vi "Slider (Main).vi"(6 "Playback":bool, 8 "Slider":i16(slide) scale=0.0..10.0, 10 "Stop":bool, 11 "Error in":errorcluster) -> (15 "Error out":errorcluster)   [LabVIEW 2020]
doc: "This system is used to playback the previous data which is needed to be plotted in the chart and the current value will also be plotted"
uses:
  Typedefs/Cluster data.ctl
panel:
  # "Dynamic and User Events"
  # "Click this button to play the previous value \nrecorded"
  # "Click this button to stop the execution of the VI"
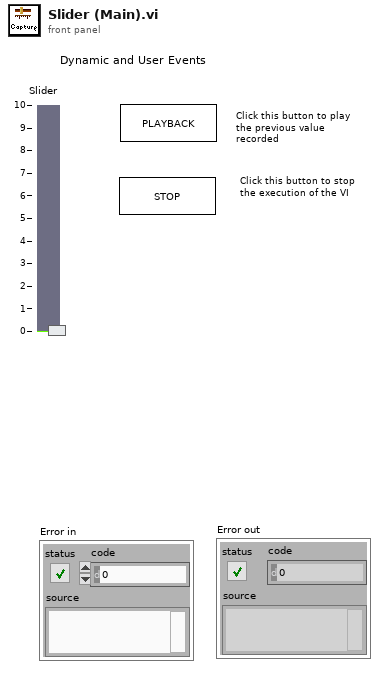
[diagram p1: front panel]
types:
  T1 = enum16{"Get Ref", "Destroy", "Create", "Generate"}
  T2 = typedef "Cluster data.ctl" = cluster{"Position":dbl, "Delay":dbl, "Boolean":bool}
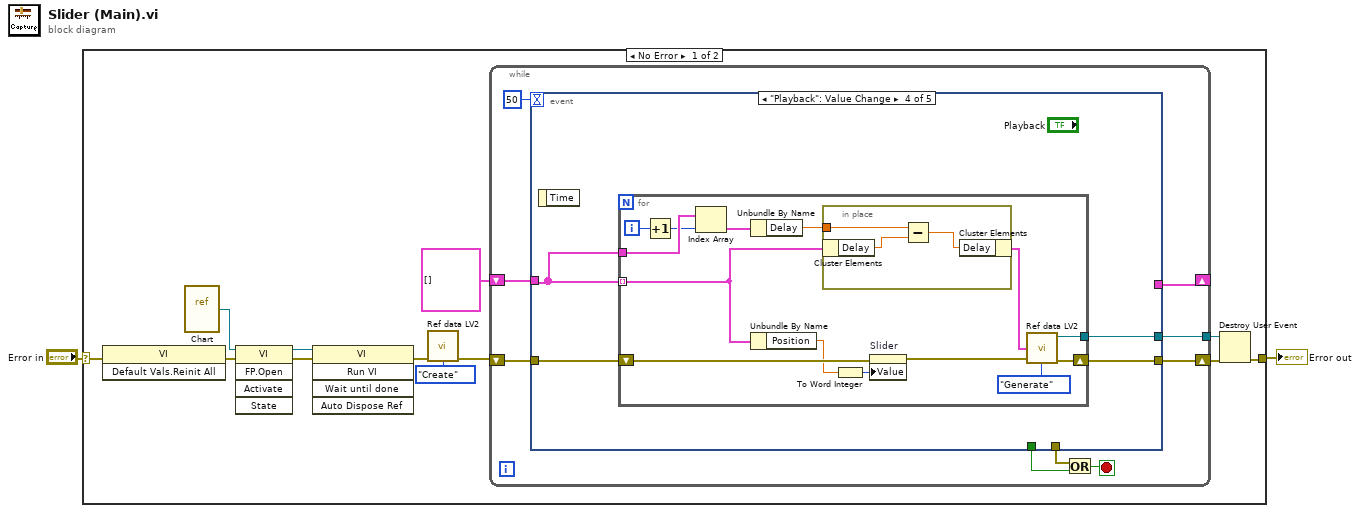
[diagram p0: block diagram]
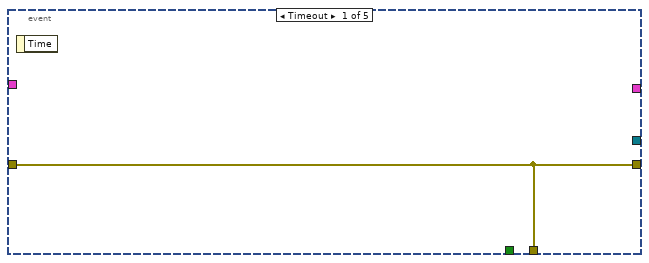
[diagram p2: hidden frame]
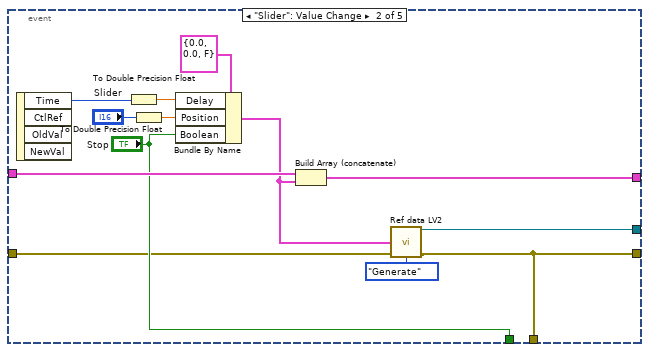
[diagram p3: hidden frame]
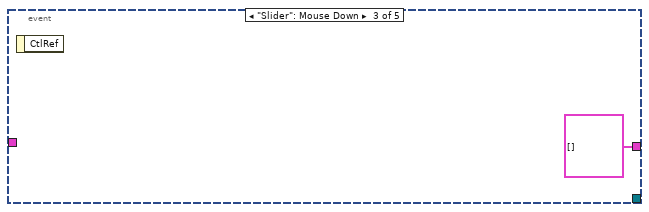
[diagram p4: hidden frame]
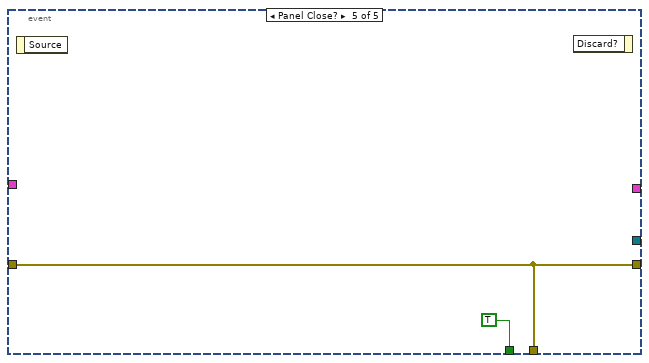
[diagram p5: hidden frame]
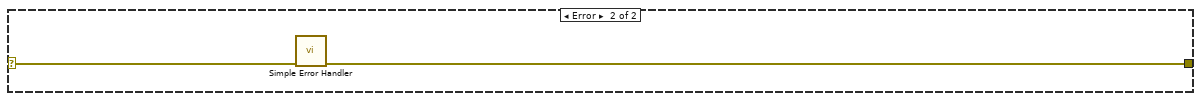
[diagram p6: hidden frame]
diagram:
  n1 = case shown="No Error" "Error in" {
    selector: "Error in" -> [w12 w63]
    tunnel: [w4 w62] -> w1
    frame No Error {
      n2 = invoke class="VI" method="Default Vals.Reinit All"(error in=w12) -> (error out=w10:errorcluster)  [unwired: 2 in, 2 out]
      n3 = vi-ref "Chart.vi"() -> (w7:refnum<vi>)
      n4 = invoke class="VI" method="FP.Open"(reference=w7, error in=w10) -> (reference out=w9:refnum<vi>, error out=w8:errorcluster)  [unwired: 3 in, 3 out]
      n5 = invoke class="VI" method="Run VI"(reference=w9, error in=w8) -> (error out=w11:errorcluster)  [unwired: 3 in, 4 out]
      n6 = call "Ref data LV2.vi"("error in"=w11, "Enum"=T1."Create") -> ("error out"=w6:errorcluster)  [unwired: 12 in, 1 out]
      n7 = while {
        shift-right: [w21] -> w5
        shift-left: w6 -> [w22]
        shift-right: [w19] -> _
        shift-left: T2[] [] -> [w18]
        tunnel: [w15] -> w3
        stop <- w20 stop-if-true
        n8 = event shown="[3] \"Playback\": Value Change" {
          selector: _ -> [_ _ _ _ _]
          dyn-events: _ -> [_ _ _ _ _]
          timeout: 50 -> [_ _ _ _ _]
          tunnel: [w24 w27 _ w40 w61] -> w21
          tunnel: w22 -> [w24 w28 _ w41 w61]
          tunnel: [_ w37 T2[] [] _ _] -> w19
          tunnel: w18 -> [_ w36 _ w42 _]
          tunnel: [w24 w27 _ _ w61] -> w17
          tunnel: [_ "Stop" _ _ TRUE ("Stop")] -> w16
          tunnel: [_ w25 _ w39 _] -> w15
          event Timeout {
            n9 = event-data() -> ()  [unwired: 1 in, 1 out]
          }
          event "Slider": Value Change {
            n10 = event-data() -> ("Time"=w31:u32)  [unwired: 1 in, 3 out]
            n11 = To Double Precision Float(number=w31) -> (double precision float=w32:dbl)
            n12 = To Double Precision Float(number="Slider") -> (double precision float=w33:dbl)
            n13 = Bundle By Name(cluster=T2 {"Position"=0.0, "Delay"=0.0, "Boolean"=FALSE} ("Data"), "Delay"=w32, "Position"=w33, "Boolean"="Stop") -> (w26:T2)
            n14 = Build Array (concatenate)(w36, w26) -> (w37:T2[])
            n15 = call "Ref data LV2.vi"("Data"=w26, "error in"=w28, "Enum"=T1."Generate") -> ("Output Refnum"=w25:refnum<user-event>, "error out"=w27:errorcluster)  [unwired: 11 in]
          }
          event "Slider": Mouse Down {
            n16 = event-data() -> ()  [unwired: 1 in, 1 out]
          }
          event "Playback": Value Change {
            n17 = event-data() -> ()  [unwired: 1 in, 1 out]
            n18 = for {
              tunnel: w42 -> [w53] mode=indexing
              tunnel: w42 -> [w55]
              shift-right: [w51] -> w40
              shift-left: w41 -> [w52]
              tunnel: [w43] -> w39
              i -> [w56]
              n19 = Increment(x=w56) -> (x+1=w54:i32)
              n20 = Index Array(array=w55, index=w54) -> (element=w50:T2)
              n21 = Unbundle By Name(w50) -> ("Delay"=w49:dbl)
              n22 = Unbundle By Name(w53) -> ("Position"=w45:dbl)
              n23 = in-place {
                in-place-border: w49 -> [w59]
                n24 = in-place-cluster #1(w53) -> ("Delay"=w58:dbl)
                n25 = Subtract(x=w59, y=w58) -> (x-y=w57:dbl)
                n26 = in-place-cluster #1("Delay"=w57) -> (w48:T2)
              }
              n27 = To Word Integer(number=w45) -> (16bit integer=w46:i16)
              n28 = property on="Slider" class="Slide (strict)"(error in=w52, "Value"=w46) -> (error out=w44:errorcluster)  [unwired: 1 in, 1 out]
              n29 = call "Ref data LV2.vi"("Data"=w48, "error in"=w44, "Enum"=T1."Generate") -> ("Output Refnum"=w43:refnum<user-event>, "error out"=w51:errorcluster)  [unwired: 11 in]
            }
          }
          event Panel Close? {
            n30 = event-data() -> ()  [unwired: 1 in, 1 out]
            n31 = event-data() -> ()  [unwired: 2 in, 1 out]
          }
        }
        n32 = Or(x=w17, y=w16) -> (x .or. y?=w20:bool)
      }
      n33 = Destroy User Event(user event=w3, error in=w5) -> (error out=w4:errorcluster)
    }
    frame Error {
      n34 = call <vilib>:"Simple Error Handler.vi"("error in (no error)"=w63) -> ("error out"=w62:errorcluster)  [unwired: 4 in, 4 out]
    }
  }
  "Error out" <- w1
